vi "SINGLE_v15_5.vi"() -> ()   [LabVIEW 2017]
uses:
  BERTTA/x64/Debug/BERTTA.dll
panel:
  in  "Add comment":string
  in  "OK Button":bool
  out "Started:":string
  in  "SHUTDOWN":bool
  in  "MASTER CONTROL":bool
  in  "Tab Control":T1(tab)
  out "Output File":path caption="selected path"
  in  "Browse folder":path=path "C:/Users/shresplab/Desktop" caption="start path"
  in  "Read Seq":bool
  in  "Save Seq":bool
  in  "Configuration file":path caption="Filename"
  in  "OK Button 2":bool
  out "Boolean":bool
  in  "User (initials)":string
  in  "Project name":string
  in  "Description":string
  out "Led11 12":bool
  out "Target amount":dbl
  out "Scale weight":dbl
  out "Amount now":dbl
  out "Flow rate":dbl
  out "Time to target":dbl format="%<%H:%M:%S>t"
  out "Current step":dbl
  out "Target":dbl
  out "Amount now":dbl
  out "PUMP3":bool
  out "Led11 11":bool
  out "Amount now":dbl
  out "Target":dbl
  out "Current step":dbl
  out "Time to target":dbl format="%<%H:%M:%S>t"
  out "Flow rate":dbl
  out "Amount now":dbl
  out "Scale weight":dbl
  out "Target amount":dbl
  out "PUMP2":bool
  out "Target amount":dbl format="Target amount:        %#_g"
  out "Scale weight":dbl format="Scale weight:     %#_4g"
  out "Amount now":dbl format="Amount now:      %#_4g"
  out "Flow rate":dbl format="Flow rate:                   %#_4g"
  out "Time to target":dbl format="Time to target:     %<%H:%M:%S>t"
  out "Current step":dbl format="Current step:              %#_g"
  out "Target":dbl format="Target:                %#_4g"
  out "Amount now":dbl format="Amount now:    %#_4g"
  out "Led11 10":bool
  out "PUMP1":bool
  out "Sensor OK 6":bool
  out "Sensor OK 5":bool
  out "Sensor OK 4":bool
  out "Sensor OK 3":bool
  out "Tr":dbl format="Tr:              %#_4g"
  out "Tj in":dbl format="Tj in:        %#_4g"
  out "Tj out":dbl format="Tj out:        %#_4g"
  out "T set":dbl format="T set:          %#_4g"
  out "Current step":i32 format="Current step:  %.0f"
  out "RPM":dbl format="RPM:          %#_g"
  out "Torque 2":dbl format="Torque:      %#_g"
  out "T external 3":dbl format="T (S2):       %#_4g"
  out "Waveform Chart 5":dynamicdata(graph)
  out "Waveform Chart 6":dynamicdata(graph)
  out "Waveform Chart 7":dynamicdata(graph)
  in  "OK Button 11":bool=TRUE
  out "Table":string[][](table)=[["14.8.2017 18.06.59", "0,000000", "417,670000", "-0,150000", "1,000000", "22,220000", "23,366837", "23,574959", "23,985852", "23,690000", "240,000000", "4,000000", "0,000000", "397,000000", "-397,000000", "1,000000"], ["14.8.2017 18.07.06", "0,000000", "417,640000", "-0,120000", "1,000000", "22,220000", "23,763115", "23,906257", "23,985694", "23,680000", "240,000000", "4,000000", "0,000000", "397,000000", "-397,000000", "1,000000"], ["14.8.2017 18.07.13", "0,000000", "417,640000", "-0,120000", "1,000000", "22,220000", "23,965922", "24,013440", "23,984906", "23,670000", "240,000000", "4,100000", "3,000000", "397,000000", "-397,000000", "1,000000"], ["14.8.2017 18.07.21", "0,000000", "417,640000", "-0,120000", "1,000000", "22,220000", "23,943860", "23,900110", "23,987113", "23,670000", "240,000000", "4,000000", "0,000000", "397,000000", "-397,000000", "1,000000"], ["14.8.2017 18.07.28", "0,000000", "417,640000", "-0,120000", "1,000000", "22,220000", "23,736328", "23,600018", "23,989004", "23,660000", "240,000000", "4,000000", "0,000000", "397,000000", "-397,000000", "1,000000"], ["14.8.2017 18.07.36", "0,000000", "417,640000", "-0,120000", "1,000000", "22,220000", "23,480910", "23,324538", "23,991053", "23,660000", "240,000000", "4,000000", "0,000000", "397,000000", "-397,000000", "1,000000"], ["14.8.2017 18.07.43", "0,000000", "417,640000", "-0,120000", "2,000000", "22,220000", "23,195579", "23,008270", "23,999093", "23,650000", "240,000000", "4,000000", "0,000000", "397,000000", "-397,000000", "1,000000"], ["14.8.2017 18.07.51", "0,000000", "417,650000", "-417,650000", "1,000000", "22,220000", "22,862541", "22,649021", "24,003979", "23,650000", "240,000000", "4,000000", "0,000000", "397,000000", "-397,000000", "2,000000"], ["14.8.2017 18.07.58", "0,000000", "417,640000", "0,010000", "1,000000", "22,220000", "22,541353", "22,354878", "24,005398", "23,650000", "240,000000", "4,000000", "0,000000", "397,000000", "-397,000000", "1,000000"], ["14.8.2017 18.08.06", "0,000000", "417,640000", "0,010000", "1,000000", "22,220000", "22,347931", "22,253738", "24,007605", "23,640000", "240,000000", "4,100000", "0,000000", "397,000000", "-397,000000", "1,000000"], ["14.8.2017 18.08.13", "0,000000", "417,640000", "0,010000", "1,000000", "22,220000", "22,329030", "22,302102", "24,006028", "23,640000", "240,000000", "4,000000", "0,000000", "395,820000", "-395,820000", "1,000000"], ["14.8.2017 18.08.20", "0,000000", "417,640000", "0,010000", "1,000000", "22,220000", "22,466849", "22,511320", "24,002403", "23,630000", "240,000000", "4,000000", "0,000000", "395,830000", "-0,010000", "1,000000"], ["14.8.2017 18.08.28", "0,000000", "417,640000", "0,010000", "1,000000", "22,220000", "22,707062", "22,835101", "24,000984", "23,620000", "240,000000", "4,000000", "0,000000", "395,830000", "-0,010000", "1,000000"], ["14.8.2017 18.08.35", "0,000000", "417,640000", "0,010000", "1,000000", "22,220000", "23,054104", "23,232979", "24,001299", "23,600000", "240,000000", "4,000000", "0,000000", "395,830000", "-0,010000", "1,000000"], ["14.8.2017 18.08.43", "0,000000", "417,640000", "0,010000", "1,000000", "22,220000", "23,412371", "23,522793", "24,002560", "23,590000", "240,000000", "4,000000", "0,000000", "395,820000", "0,000000", "1,000000"], ["14.8.2017 18.08.51", "0,000000", "417,640000", "0,010000", "1,000000", "22,220000", "23,596247", "23,656125", "24,003821", "23,580000", "240,000000", "4,000000", "0,000000", "395,820000", "0,000000", "1,000000"]]
  out "LED_5":bool
  out "LED_4":bool
  in  "PAUSE/RUN 4":bool
  in  "TEMP RAMP":dbl[][](array[numeric])
  out "LED_3":bool
  out "LED_2":bool
  out "LED_1":bool
  out "LED_MANUAL":bool
  in  "Reset 6":bool
  in  "Manual/Ramp":bool=TRUE
  in  "Sensor selector":bool=TRUE
  in  "Tr/Tj mode selector":bool=TRUE
  out "LED STOP":bool
  in  "Failsafe":dbl=20.0 format="Failsafe temperature:            %#_g"
  out "Current temp":dbl format="Current temperature S1:       %#_4g"
  out "Sensor OK":bool
  out "T external 2":dbl format="Current temperature S2:       %#_4g"
  in  "OK Button 3":bool
  out "Waveform Chart":dynamicdata(graph)
  in  "X scales":i64(slide)=50 scale=0.0..100.0
  in  "PAUSE/RUN 9":bool=TRUE
  out "Led11 7":bool
  out "Led11 6":bool
  in  "PAUSE/RUN 3":bool
  in  "Tube select 3":u32(ring) items=["Big tube", "Double big tube", "Medium tube", "Small tube"]
  in  "Reset 8":bool
  out "Led11 9":bool
  in  "?":bool
  in  "Grams / min 3":dbl
  out "RPM 3":dbl format="%_4f"
  out "Flow rate (g/min) 3":dbl
  out "Scale reading 3":dbl
  out "Step amount now 3":dbl
  out "Total amount now 3":dbl
  out "Elapsed / step 3":dbl format="%<%H:%M:%S>t"
  out "Time to target 3":dbl format="%<%H:%M:%S>t"
  out "Led5 5":bool
  out "Led4 5":bool
  out "Led3 5":bool
  out "Led2 5":bool
  out "Led1 5":bool
  in  "PumpSeq 6":dbl[][](array[numeric])=[[0.0, 0.0, 0.0, 0.0, 0.0, 0.0, 0.0, 0.0, 0.0, 0.0], [0.0, 0.0, 0.0, 0.0, 0.0, 0.0, 0.0, 0.0, 0.0, 0.0], [0.0, 0.0, 0.0, 0.0, 0.0, 0.0, 0.0, 0.0, 0.0, 0.0], [0.0, 0.0, 0.0, 0.0, 0.0, 0.0, 0.0, 0.0, 0.0, 0.0], [0.0, 0.0, 0.0, 0.0, 0.0, 0.0, 0.0, 0.0, 0.0, 0.0], [0.0, 0.0, 0.0, 0.0, 0.0, 0.0, 0.0, 0.0, 0.0, 0.0], [0.0, 0.0, 0.0, 0.0, 0.0, 0.0, 0.0, 0.0, 0.0, 0.0], [0.0, 0.0, 0.0, 0.0, 0.0, 0.0, 0.0, 0.0, 0.0, 0.0], [0.0, 0.0, 0.0, 0.0, 0.0, 0.0, 0.0, 0.0, 0.0, 0.0], [0.0, 0.0, 0.0, 0.0, 0.0, 0.0, 0.0, 0.0, 0.0, 0.0]]
  out "Led11 8":bool
  in  "PAUSE/RUN 8":bool=TRUE
  out "Led11 7":bool
  out "Led11 6":bool
  in  "PAUSE/RUN 2":bool
  in  "Tube select 2":u32(ring) items=["Big tube", "Double big tube", "Medium tube", "Small tube"]
  out "Led11 7":bool
  in  "?":bool
  in  "Grams / min 2":dbl
  out "RPM 2":dbl format="%_4f"
  out "Flow rate (g/min) 2":dbl
  out "Scale reading 2":dbl
  out "Step amount now 2":dbl
  out "Total amount now 2":dbl
  out "Elapsed / step 2":dbl format="%<%H:%M:%S>t"
  out "Time to target 2":dbl format="%<%H:%M:%S>t"
  out "Led5 4":bool
  out "Led4 4":bool
  out "Led3 4":bool
  out "Led2 4":bool
  out "Led1 4":bool
  in  "PumpSeq 5":dbl[][](array[numeric])=[[0.0, 0.0, 0.0, 0.0, 0.0, 0.0, 0.0, 0.0, 0.0, 0.0], [0.0, 0.0, 0.0, 0.0, 0.0, 0.0, 0.0, 0.0, 0.0, 0.0], [0.0, 0.0, 0.0, 0.0, 0.0, 0.0, 0.0, 0.0, 0.0, 0.0], [0.0, 0.0, 0.0, 0.0, 0.0, 0.0, 0.0, 0.0, 0.0, 0.0], [0.0, 0.0, 0.0, 0.0, 0.0, 0.0, 0.0, 0.0, 0.0, 0.0], [0.0, 0.0, 0.0, 0.0, 0.0, 0.0, 0.0, 0.0, 0.0, 0.0], [0.0, 0.0, 0.0, 0.0, 0.0, 0.0, 0.0, 0.0, 0.0, 0.0], [0.0, 0.0, 0.0, 0.0, 0.0, 0.0, 0.0, 0.0, 0.0, 0.0], [0.0, 0.0, 0.0, 0.0, 0.0, 0.0, 0.0, 0.0, 0.0, 0.0], [0.0, 0.0, 0.0, 0.0, 0.0, 0.0, 0.0, 0.0, 0.0, 0.0]]
  out "Led11 6":bool
  in  "Reset 7":bool
  in  "PAUSE/RUN 7":bool=TRUE
  out "Led5 7":bool
  out "Led4 6":bool
  in  "PAUSE/RUN":bool
  in  "Tube select":u32(ring) items=["Big tube", "Double big tube", "Medium tube", "Small tube"]
  out "Led11 5":bool
  out "RPM":dbl format="RPM                      %_4f"
  out "Flow rate (g/min)":dbl format="Flow rate               %#_g"
  out "Scale reading":dbl format="Scale reading       %#_g"
  out "Step amount now":dbl format="Step amount       %#_g"
  out "Total amount now":dbl format="Total amount      %#_g"
  out "Elapsed / step":dbl format="Elapsed / step      %<%H:%M:%S>t"
  out "Time to target":dbl format="Time to target     %<%H:%M:%S>t"
  out "Led5 3":bool
  out "Led4 3":bool
  out "Led3 3":bool
  out "Led2 3":bool
  out "Led1 3":bool
  in  "PumpSeq 4":dbl[][](array[numeric])=[[0.0, 0.0, 0.0, 0.0, 0.0, 0.0, 0.0, 0.0, 0.0, 0.0], [0.0, 0.0, 0.0, 0.0, 0.0, 0.0, 0.0, 0.0, 0.0, 0.0], [0.0, 0.0, 0.0, 0.0, 0.0, 0.0, 0.0, 0.0, 0.0, 0.0], [0.0, 0.0, 0.0, 0.0, 0.0, 0.0, 0.0, 0.0, 0.0, 0.0], [0.0, 0.0, 0.0, 0.0, 0.0, 0.0, 0.0, 0.0, 0.0, 0.0], [0.0, 0.0, 0.0, 0.0, 0.0, 0.0, 0.0, 0.0, 0.0, 0.0], [0.0, 0.0, 0.0, 0.0, 0.0, 0.0, 0.0, 0.0, 0.0, 0.0], [0.0, 0.0, 0.0, 0.0, 0.0, 0.0, 0.0, 0.0, 0.0, 0.0], [0.0, 0.0, 0.0, 0.0, 0.0, 0.0, 0.0, 0.0, 0.0, 0.0], [0.0, 0.0, 0.0, 0.0, 0.0, 0.0, 0.0, 0.0, 0.0, 0.0]]
  in  "?":bool
  in  "Grams / min":dbl format="Manual g/min:  %#_g"
  out "Led11 4":bool
  in  "Reset 5":bool
  out "Waveform Chart 18":dynamicdata(graph)
  in  "OK Button 4":bool
  out "Waveform Chart 16":dynamicdata(graph)
  in  "OK Button 5":bool
  out "Waveform Chart 17":dynamicdata(graph)
  in  "OK Button 6":bool
  in  "PAUSE/RUN 5":bool
  in  "?":bool
  in  "Scale port":dbl=5.0
  out "Waveform Chart 15":dynamicdata(graph)
  in  "OK Button 8":bool
  in  "PAUSE/RUN 6":bool
  in  "Set RPM":i32
  in  "Remote / Manual":bool
  out "RPM":dbl
  out "Torque":dbl
  out "Waveform Chart 4":dynamicdata(graph)
  in  "OK Button 7":bool
  in  "CDAQ 1 Temp Control":tag="EASY9217_1"
  in  "CDAQ PAM Control":tag="EASY9747"
  in  "PORT PUMP2":i32 format="PUMP 2 PORT:  %.0f"
  in  "PORT PUMP3":i32 format="PUMP 3 PORT:  %.0f"
  in  "PORT PUMP1":i32 format="PUMP 1 PORT:  %.0f"
  in  "Save PortDev":bool
  in  "LAUDA":i32 format="LAUDA 1 PORT:  %.0f"
  in  "HEIDOLPH":i32 format="HEIDOLPH 1 PORT:  %.0f"
  in  "SCALE1":i32 format="SCALE 1 PORT:  %.0f"
  in  "SCALE2":i32 format="SCALE 2 PORT:  %.0f"
  in  "SCALE 3":i32 format="SCALE 3 PORT:  %.0f"
  # "Sensor:"
  # "Control:"
  # "PUMP & SCALE 3"
  # "STEP"
  # "TOTAL"
  # "PUMP & SCALE 2"
  # "STEP"
  # "TOTAL"
  # "PUMP & SCALE 1"
  # "STEP"
  # "TOTAL"
  # "MANUAL"
  # "RAMP"
  # "Temp Target       Time Target          Wait Time"
  # "STOP"
  # "g              min"
  # "g              min"
  # "g              min"
  # "PAM control"
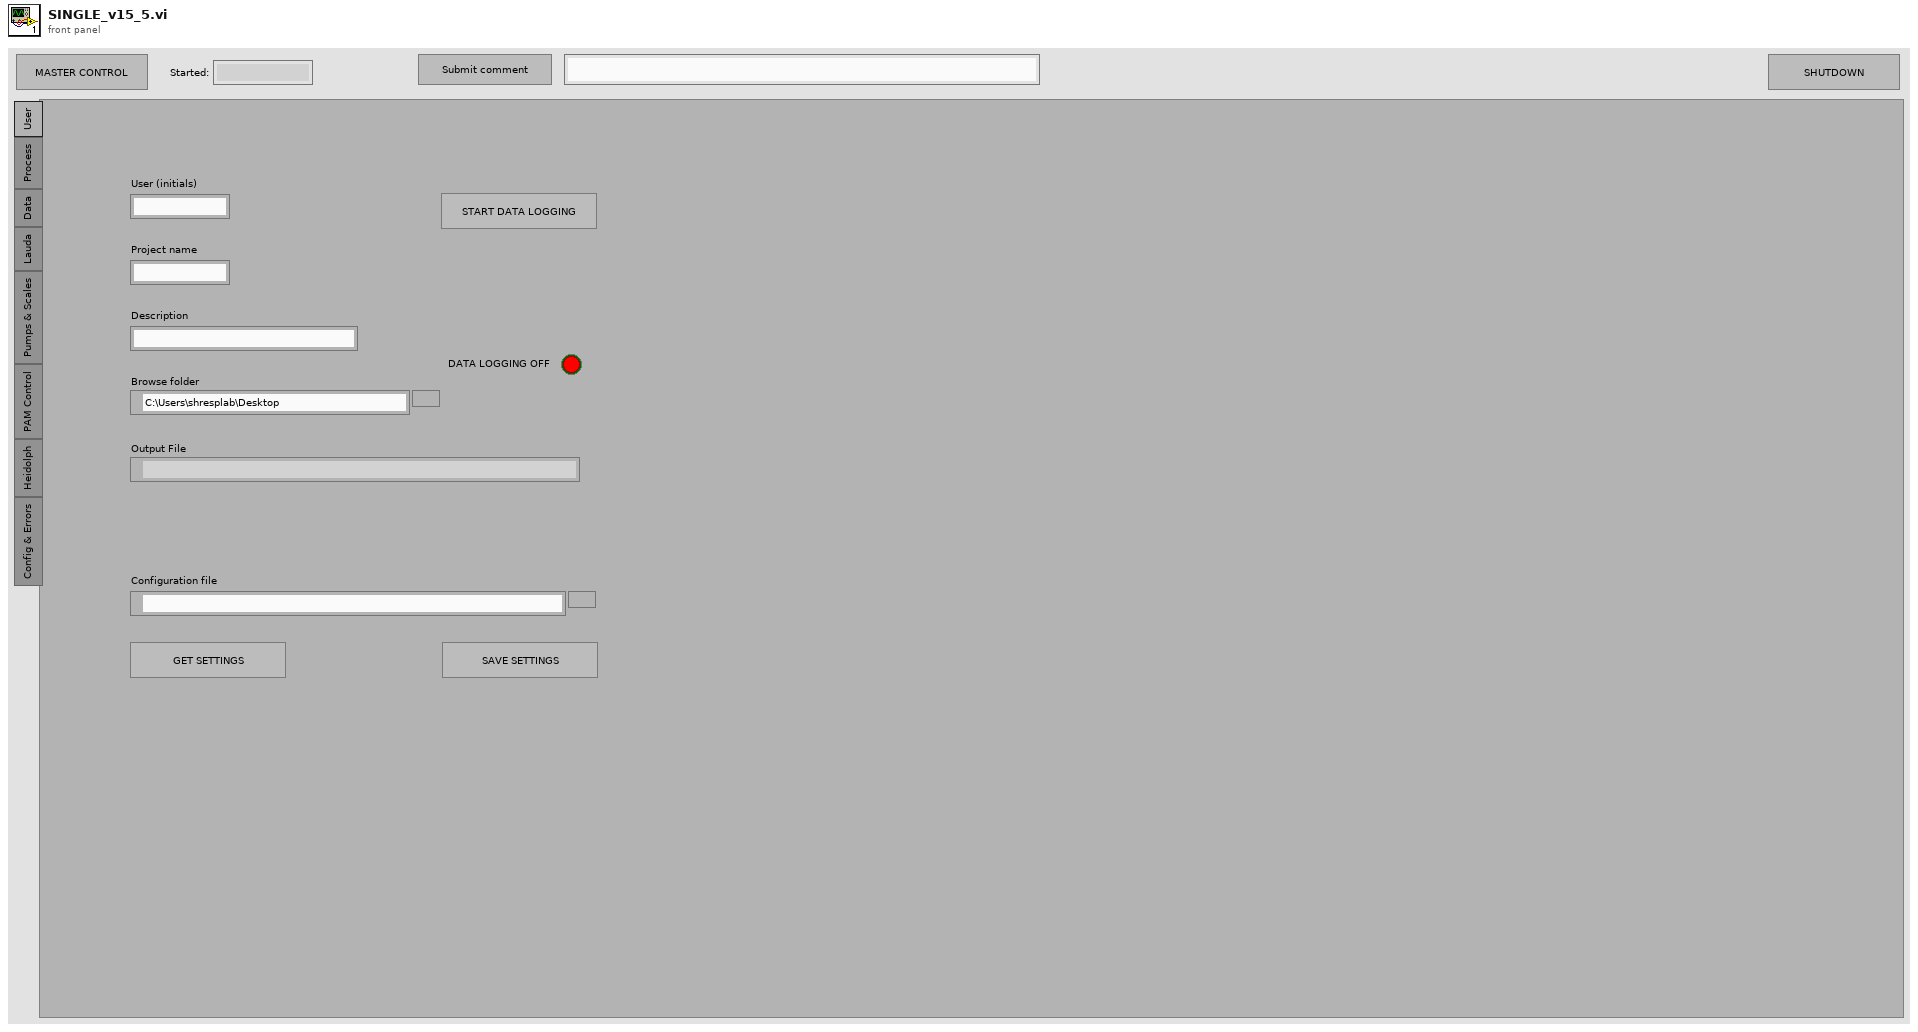
[diagram p1: front panel]
types:
  T1 = enum32{"User", "Process", "Data", "Lauda", "Pumps & Scales", "PAM Control", "Heidolph", "Config & Errors"}
diagram:
  n1 = while {
    i -> [w192]
    stop <- FALSE stop-if-true
    w126 = i64 1000 ("y")
    # "SCALE & PUMP 3"
    n2 = And(x="PAUSE/RUN 6", y="MASTER CONTROL") -> (x .and. y?=w116:bool)
    n3 = Not(x="MASTER CONTROL") -> (.not. x?=w227:bool)
    n4 = Boolean To (0,1)(Boolean="PAUSE/RUN 7") -> (0, 1=w12:i16)
    n5 = Boolean To (0,1)(Boolean="PAUSE/RUN 8") -> (0, 1=w11:i16)
    n6 = Boolean To (0,1)(Boolean="PAUSE/RUN 9") -> (0, 1=w10:i16)
    n7 = control-ref of="This VI"() -> (w112:refnum<vi>)
    n8 = Multiply(x="X scales", y=w126) -> (x*y=w127:i64)
    n9 = Boolean To (0,1)(Boolean=w227) -> (0, 1=w228:i16)
    n10 = call "RampCTRL_1.vi"("TEMP RAMP"="TEMP RAMP", "Reset 6"="Reset 6") -> ("Array"=w149:dbl[], "Array 2"=w150:dbl[], "Array 3"=w151:dbl[])  [unwired: 7 in]
    n11 = Add(x=w127, y=w126) -> (x+y=w32:i64)
    n12 = for {
      N: w228 -> [_]
      n13 = Get Date/Time String(want seconds? (F)=TRUE) -> (time string=→"Started:":string)  [unwired: 2 in, 1 out]
    }
    n14 = Select(t="Set RPM", s=w116, f=10) -> (s? t:f=w119:i32)
    n15 = Boolean To (0,1)(Boolean="Sensor selector") -> (0, 1=w144:i16)
    n16 = feedback #1() -> (w125:i64)  [unwired: 1 in]
    n17 = feedback-in #1(w32) -> ()
    n18 = call "shutdown sequence.vi"("SHUTDOWN"="SHUTDOWN", "VI in"=w112) -> ()  [unwired: 10 in]
    n19 = Boolean To (0,1)(Boolean="SHUTDOWN") -> (0, 1=w111:i16)
    n20 = Boolean To (0,1)(Boolean="Reset 6") -> (0, 1=w161:i16)
    n21 = Not Equal?(x=w125, y=w32) -> (x != y?=w124:bool)
    n22 = property on="Waveform Chart" class="WFChart (strict)"() -> ("History Data"=w129:dynamicdata[])  [unwired: 2 in, 2 out]
    n23 = Boolean To (0,1)(Boolean="SHUTDOWN") -> (0, 1=w113:i16)
    n24 = Boolean To (0,1)(Boolean=w124) -> (0, 1=w122:i16)
    n25 = Array Size(array=w129) -> (size(s)=w123:i32)
    n26 = call "ReadMoxa8.vi"("PORT 1"="LAUDA", "PORT 2"="HEIDOLPH", "PORT 3"="SCALE1", "PORT 4"="SCALE2", "PORT 5"="SCALE 3", "PORT 6"="PORT PUMP1", "PORT 7"="PORT PUMP2", "PORT 8"="PORT PUMP3", "enable1"=w12, "enable2"=w11, "enable3"=w10) -> ("params"=w14:dbl[])  [unwired: 8 in]
    n27 = call "HEI_CTRL.vi"("shutdown"=w113, "Set RPM"=w119, "Remote / Manual"="Remote / Manual", "port3"="HEIDOLPH") -> ()  [unwired: 8 in]
    n28 = Boolean To (0,1)(Boolean="Tr/Tj mode selector") -> (0, 1=w145:i16)
    n29 = call "SensorMode1.vi"("Numeric"=w144, "Numeric 2"=w145) -> ("Sensor OK 4"=→"Sensor OK 4":bool, "Sensor OK 5"=→"Sensor OK 5":bool, "Sensor OK 6"=→"Sensor OK 6":bool, "Sensor OK 3"=→"Sensor OK 3":bool)  [unwired: 6 in]
    n30 = for {
      N: w122 -> [_]
      tunnel: w123 -> [w241]
      tunnel: w32 -> [w240]
      n31 = Add(x=w241, y=w240) -> (x+y=w239:i64)
      n32 = property on="Waveform Chart" class="WFChart (strict)"("XScale.Maximum"=w239) -> ()  [unwired: 2 in, 2 out]
    }
    n33 = Boolean To (0,1)(Boolean="Manual/Ramp") -> (0, 1=w159:i16)
    n34 = And(x="MASTER CONTROL", y="PAUSE/RUN 4") -> (x .and. y?=w158:bool)
    n35 = Build Array("LAUDA", "HEIDOLPH", "SCALE1", "SCALE2", "SCALE 3", "PORT PUMP1", "PORT PUMP2", "PORT PUMP3") -> (w133:i32[])
    n36 = Boolean To (0,1)(Boolean=w158) -> (0, 1=w157:i16)
    n37 = call "LaudaDAQ.vi"("device name"="CDAQ 1 Temp Control") -> (1:"Tj out"=→"Tj out":dbl, "data"=w221:dynamicdata, "Sensor OK"=→"Sensor OK":bool, 4:"Tj out"=→"Tj in":dbl, "T external 2"=w115:dbl)  [unwired: 5 in, 1 out]
    "T external 2" <- w115
    "T external 3" <- w115
    n38 = call "Ramp_Lauda_v3.vi"("manual"=w159, "Tr_Tj"=w145, "shutdown"=w111, "S1_S2"=w144, "Tr"=w14, "T_fail"="Failsafe", "enable"=w157, "time_set"=w150, "reset"=w161, "time_wait"=w149, "T_S2"=w115, "port"="LAUDA", "T_sp"=w151) -> ("LED_1"=→"LED_1":bool, "LED_manual"=→"LED_MANUAL":bool, "LED_2"=→"LED_2":bool, "step"=w136:dbl, "LED_stop"=→"LED STOP":bool, "LED_3"=→"LED_3":bool, "LED 4"=→"LED_4":bool, "LED 5"=→"LED_5":bool, "setpoint"=w15:dbl, "Tr_out"=w156:dbl, "T int"=w155:dbl)  [unwired: 2 in, 2 out]
    "Tr" <- w156
    "T set" <- w15
    "Current temp" <- w156
    n39 = Boolean To (0,1)(Boolean="Save PortDev") -> (0, 1=w195:i16)
    n40 = for {
      N: w195 -> [_]
      tunnel: w133 -> [w287]
      tunnel: "Save PortDev" -> [w288]
      n41 = call "Convert to Dynamic Data"("Array"=w287) -> ("Dynamic Data Type"=w286:dynamicdata)  [unwired: 3 in]
      n42 = call "Write To Measurement File3"("Signals"=w286, "Reset"=w288) -> ()  [unwired: 15 in, 3 out]
    }
    n43 = Add(x=w136, y=1.0) -> (x+y=→"Current step":dbl)
    n44 = Merge Signals(w15, w156, w155, w221) -> (w22:dynamicdata)
    "Waveform Chart" <- w22
    "Waveform Chart 5" <- w22
    n45 = Less?(x=w192, y=1.0) -> (x < y?=w190:bool)
    n46 = call "HEI_Data_single.vi"("params"=w14) -> ("RPM"=→"RPM" →"RPM":dbl, "Dynamic Data"=w26:dynamicdata, "Torque 2"=→"Torque 2":dbl, "Waveform Chart 4"=→"Waveform Chart 4":dynamicdata, "Torque"=→"Torque":dbl, "Waveform Chart 6"=→"Waveform Chart 6":dynamicdata)  [unwired: 12 in, 1 out]
    n47 = Boolean To (0,1)(Boolean=w190) -> (0, 1=w191:i16)
    n48 = for {
      N: w191 -> [_]
      tunnel: w190 -> [w281]
      n49 = while {
        tunnel: [w284] -> w280
        tunnel: w281 -> [w282]
        stop <- w285 stop-if-true
        n50 = call "Read From Measurement File2"("Enable"=TRUE, "Reset"=w282) -> ("Signals"=w284:dynamicdata, "EOF?"=w285:bool)  [unwired: 4 in, 4 out]
      }
      n51 = call "Convert from Dynamic Data2"("Dynamic Data Type"=w280) -> ("Array"=w263:dbl[])  [unwired: 3 in]
      n52 = Index Array(array=w263, index=0) -> (element=w273:dbl)
      n53 = Index Array(array=w263, index=1) -> (element=w272:dbl)
      n54 = Index Array(array=w263, index=2) -> (element=w271:dbl)
      n55 = Index Array(array=w263, index=3) -> (element=w270:dbl)
      n56 = Index Array(array=w263, index=4) -> (element=w269:dbl)
      n57 = Index Array(array=w263, index=5) -> (element=w264:dbl)
      n58 = Index Array(array=w263, index=6) -> (element=w266:dbl)
      n59 = Index Array(array=w263, index=7) -> (element=w265:dbl)
      n60 = property on="LAUDA" class="DigNum (strict)"("Val(Sgnl)"=w273) -> ()  [unwired: 2 in, 2 out]
      n61 = property on="HEIDOLPH" class="DigNum (strict)"("Val(Sgnl)"=w272) -> ()  [unwired: 2 in, 2 out]
      n62 = property on="SCALE1" class="DigNum (strict)"("Val(Sgnl)"=w271) -> ()  [unwired: 2 in, 2 out]
      n63 = property on="SCALE2" class="DigNum (strict)"("Val(Sgnl)"=w270) -> ()  [unwired: 2 in, 2 out]
      n64 = property on="SCALE 3" class="DigNum (strict)"("Val(Sgnl)"=w269) -> ()  [unwired: 2 in, 2 out]
      n65 = property on="PORT PUMP1" class="DigNum (strict)"("Val(Sgnl)"=w264) -> ()  [unwired: 2 in, 2 out]
      n66 = property on="PORT PUMP2" class="DigNum (strict)"("Val(Sgnl)"=w266) -> ()  [unwired: 2 in, 2 out]
      n67 = property on="PORT PUMP3" class="DigNum (strict)"("Val(Sgnl)"=w265) -> ()  [unwired: 2 in, 2 out]
    }
    n68 = Boolean To (0,1)(Boolean="OK Button 3") -> (0, 1=w202:i16)
    n69 = for {
      N: w202 -> [_]
      n70 = property on="Waveform Chart" class="WFChart (strict)"("History Data"=dynamicdata[] []) -> ()  [unwired: 2 in, 2 out]
    }
    n71 = Boolean To (0,1)(Boolean="OK Button 4") -> (0, 1=w200:i16)
    n72 = for {
      N: w200 -> [_]
      n73 = property on="Waveform Chart 18" class="WFChart (strict)"("History Data"=dynamicdata[] []) -> ()  [unwired: 2 in, 2 out]
    }
    n74 = Boolean To (0,1)(Boolean="OK Button 5") -> (0, 1=w142:i16)
    n75 = for {
      N: w142 -> [_]
      n76 = property on="Waveform Chart 16" class="WFChart (strict)"("History Data"=dynamicdata[] []) -> ()  [unwired: 2 in, 2 out]
    }
    n77 = call "IsmaCTRL_single.vi"("FR_manual"="Grams / min", "tube selector"="Tube select", "Manual"="?", "Reset"="Reset 5", "Pause"="PAUSE/RUN", "Setpoint_W   /   Setpoint_T"="PumpSeq 4", "Enable"="MASTER CONTROL", "Scale"=w14) -> ("Boolean 9"=→"Led11 5" →"Led11 10":bool, "Boolean"=→"Led1 3":bool, "Boolean 2"=→"Led2 3":bool, "Total target"=→"Target":dbl, "Boolean 3"=→"Led3 3":bool, "Boolean 4"=→"Led4 3":bool, "lastAmount"=→"Step amount now":dbl, "step"=→"Current step":dbl, "Boolean 5"=→"Led5 3":bool, "Boolean 6"=→"Led4 6":bool, "Boolean 7"=→"Led5 7":bool, "FR"=w94:dbl, "RPM"=w18:dbl, "Weight"=w90:dbl, "elapsed"=→"Elapsed / step":dbl, "time_to_target"=→"Time to target" →"Time to target":dbl, "pumpCTRL"=w106:dbl, "Target_step"=→"Target amount":dbl, "Boolean 8"=w98:bool)  [unwired: 1 out]
    "Flow rate" <- w94
    "Scale weight" <- w90
    "Led11 4" <- w98
    "Scale reading" <- w90
    "Flow rate (g/min)" <- w94
    "RPM" <- w18
    n78 = Boolean To (0,1)(Boolean="OK Button 6") -> (0, 1=w140:i16)
    n79 = for {
      N: w140 -> [_]
      n80 = property on="Waveform Chart 17" class="WFChart (strict)"("History Data"=dynamicdata[] []) -> ()  [unwired: 2 in, 2 out]
    }
    n81 = Multiply(x=w90, y=-1.0 ("x")) -> (x*y=→"Amount now" →"Amount now" →"Total amount now":dbl)
    n82 = And(x="PAUSE/RUN", y=w98) -> (x .and. y?=w178:bool)
    n83 = feedback #2() -> (w179:bool)  [unwired: 1 in]
    n84 = feedback-in #2(w178) -> ()
    n85 = Greater?(x=w106, y=70.0) -> (0:→"PUMP1":bool)
    n86 = Not Equal?(x=w179, y=w178) -> (x != y?=w177:bool)
    n87 = Boolean To (0,1)(Boolean=w177) -> (0, 1=w176:i16)
    n88 = for {
      N: w176 -> [_]
      n89 = property on="PAUSE/RUN" class="Bool (strict)"("Val(Sgnl)"=FALSE ("Value (Signaling)")) -> ()  [unwired: 2 in, 2 out]
    }
    n90 = Merge Signals(w90, w94) -> (w143:dynamicdata)
    "Waveform Chart 18" <- w143
    n91 = Boolean To (0,1)(Boolean="OK Button 7") -> (0, 1=w198:i16)
    n92 = for {
      N: w198 -> [_]
      n93 = property on="Waveform Chart 4" class="WFChart (strict)"("History Data"=dynamicdata[] []) -> ()  [unwired: 2 in, 2 out]
    }
    n94 = call "IsmaCTRL_2_single.vi"("FR_manual"="Grams / min 2", "tube selector"="Tube select 2", "Manual"="?", "Reset"="Reset 7", "Pause"="PAUSE/RUN 2", "Setpoint_W   /   Setpoint_T"="PumpSeq 5", "Enable"="MASTER CONTROL", "Scale"=w14) -> ("Boolean 9"=→"Led11 7" →"Led11 11":bool, "Boolean"=→"Led1 4":bool, "Boolean 2"=→"Led2 4":bool, "Total target"=→"Target":dbl, "Boolean 3"=→"Led3 4":bool, "Boolean 4"=→"Led4 4":bool, "lastAmount"=→"Amount now" →"Step amount now 2":dbl, "step"=→"Current step":dbl, "Boolean 5"=→"Led5 4":bool, "Boolean 6"=→"Led11 6":bool, "Boolean 7"=→"Led11 7":bool, "FR"=w77:dbl, "RPM"=w17:dbl, "Weight"=w78:dbl, "elapsed"=→"Elapsed / step 2":dbl, "time_to_target"=→"Time to target" →"Time to target 2":dbl, "pumpCTRL"=w71:dbl, "Target_step"=→"Target amount":dbl, "Boolean 8"=w61:bool)  [unwired: 1 out]
    "Scale weight" <- w78
    "Flow rate" <- w77
    "Led11 6" <- w61
    "Scale reading 2" <- w78
    "Flow rate (g/min) 2" <- w77
    "RPM 2" <- w17
    n95 = Boolean To (0,1)(Boolean="OK Button 8") -> (0, 1=w185:i16)
    n96 = for {
      N: w185 -> [_]
      n97 = property on="Waveform Chart 15" class="WFChart (strict)"("History Data"=dynamicdata[] []) -> ()  [unwired: 2 in, 2 out]
    }
    n98 = Merge Signals(w78, w77) -> (w173:dynamicdata)
    "Waveform Chart 16" <- w173
    n99 = Multiply(x=w78, y=-1.0) -> (x*y=→"Amount now" →"Total amount now 2":dbl)
    n100 = And(x="PAUSE/RUN 2", y=w61) -> (x .and. y?=w171:bool)
    n101 = Greater?(x=w71, y=70.0) -> (0:→"PUMP2":bool)
    n102 = feedback #3() -> (w172:bool)  [unwired: 1 in]
    n103 = feedback-in #3(w171) -> ()
    n104 = Not Equal?(x=w172, y=w171) -> (x != y?=w170:bool)
    n105 = Boolean To (0,1)(Boolean=w170) -> (0, 1=w169:i16)
    n106 = for {
      N: w169 -> [_]
      n107 = property on="PAUSE/RUN 2" class="Bool (strict)"("Val(Sgnl)"=FALSE ("Value (Signaling)")) -> ()  [unwired: 2 in, 2 out]
    }
    n108 = call "IsmaCTRL_3_single.vi"("FR_manual"="Grams / min 3", "tube selector"="Tube select 3", "Manual"="?", "Reset"="Reset 8", "Pause"="PAUSE/RUN 3", "Setpoint_W   /   Setpoint_T"="PumpSeq 6", "Enable"="MASTER CONTROL", "Scale"=w14) -> ("Boolean 9"=→"Led11 9" →"Led11 12":bool, "Boolean"=→"Led1 5":bool, "Boolean 2"=→"Led2 5":bool, "Total target"=→"Target":dbl, "Boolean 3"=→"Led3 5":bool, "Boolean 4"=→"Led4 5":bool, "lastAmount"=→"Amount now" →"Step amount now 3":dbl, "step"=→"Current step":dbl, "Boolean 5"=→"Led5 5":bool, "Boolean 6"=→"Led11 6":bool, "Boolean 7"=→"Led11 7":bool, "FR"=w47:dbl, "RPM"=w16:dbl, "Weight"=w46:dbl, "elapsed"=→"Elapsed / step 3":dbl, "time_to_target"=→"Time to target" →"Time to target 3":dbl, "pumpCTRL"=w52:dbl, "Target_step"=→"Target amount":dbl, "Boolean 8"=w37:bool)  [unwired: 1 out]
    "Scale weight" <- w46
    "Flow rate" <- w47
    "Led11 8" <- w37
    "Scale reading 3" <- w46
    "Flow rate (g/min) 3" <- w47
    "RPM 3" <- w16
    n109 = call "WriteMoxa8.vi"("PORT LAUDA 1"="LAUDA", "DATA LAUDA 1"=w15, "enable2"=w11, "DATA ISMA 1"=w18, "DATA ISMA 2"=w17, "enable1"=w12, "PORT ISMA 1"="PORT PUMP1", "DATA ISMA 3"=w16, "PORT ISMA 2"="PORT PUMP2", "PORT ISMA 3"="PORT PUMP3", "enable3"=w10) -> ()  [unwired: 5 in]
    n110 = Multiply(x=w46, y=-1.0) -> (x*y=→"Amount now" →"Total amount now 3":dbl)
    n111 = Merge Signals(w90, w78, w46) -> (→"Waveform Chart 7":dynamicdata)
    n112 = Greater?(x=w52, y=70.0) -> (0:→"PUMP3":bool)
    n113 = And(x="MASTER CONTROL", y=w37) -> (x .and. y?=w164:bool)
    n114 = Merge Signals(w46, w47) -> (w166:dynamicdata)
    "Waveform Chart 17" <- w166
    n115 = feedback #4() -> (w165:bool)  [unwired: 1 in]
    n116 = feedback-in #4(w164) -> ()
    n117 = Not Equal?(x=w165, y=w164) -> (x != y?=w163:bool)
    n118 = Boolean To (0,1)(Boolean=w163) -> (0, 1=w162:i16)
    n119 = for {
      N: w162 -> [_]
      n120 = property on="PAUSE/RUN 3" class="Bool (strict)"("Val(Sgnl)"=FALSE ("Value (Signaling)")) -> ()  [unwired: 2 in, 2 out]
    }
    n121 = call "Convert to Dynamic Data6"() -> ("Dynamic Data Type"=w21:dynamicdata)  [unwired: 4 in]
    n122 = call "Convert to Dynamic Data4"("2D Array"="PumpSeq 6") -> ("Dynamic Data Type"=w208:dynamicdata)  [unwired: 3 in]
    n123 = call "Convert to Dynamic Data3"("2D Array"="PumpSeq 5") -> ("Dynamic Data Type"=w209:dynamicdata)  [unwired: 3 in]
    n124 = call "Convert to Dynamic Data2"("2D Array"="PumpSeq 4") -> ("Dynamic Data Type"=w211:dynamicdata)  [unwired: 3 in]
    n125 = Merge Signals(w21, w208, w209, w211) -> (w210:dynamicdata)
    n126 = Boolean To (0,1)(Boolean="Save Seq") -> (0, 1=w207:i16)
    n127 = for {
      N: w207 -> [_]
      tunnel: w210 -> [w320]
      tunnel: "Configuration file" -> [w321]
      tunnel: "Save Seq" -> [w319]
      n128 = call "Write To Measurement File2"("Signals"=w320, "Reset"=w319, "Filename"=w321) -> ()  [unwired: 14 in, 3 out]
    }
    n129 = Boolean To (0,1)(Boolean="Read Seq") -> (0, 1=w206:i16)
    n130 = for {
      N: w206 -> [_]
      tunnel: "Configuration file" -> [w306]
      tunnel: "Read Seq" -> [w305]
      n131 = while {
        tunnel: [w318] -> w314
        tunnel: w306 -> [w317]
        tunnel: w305 -> [w315]
        stop <- w316 stop-if-true
        n132 = call "Read From Measurement File"("Filename"=w317, "Reset"=w315) -> ("Signals"=w318:dynamicdata, "EOF?"=w316:bool)  [unwired: 4 in, 4 out]
      }
      n133 = call "Convert from Dynamic Data"("Dynamic Data Type"=w314) -> ("Array"=w309:dbl[][])  [unwired: 3 in]
      n134 = Array Subset(array=w309, index (row)=20 ("index"), length (row)=10 ("length")) -> (w302:dbl[][])  [unwired: 2 in]
      n135 = Array Subset(array=w309, index (row)=10 ("index"), length (row)=10 ("length")) -> (w303:dbl[][])  [unwired: 2 in]
      n136 = Array Subset(array=w309, index (row)=30 ("index"), length (row)=8 ("length")) -> (w304:dbl[][])  [unwired: 2 in]
      n137 = property on="PumpSeq 6" class="Arr (strict)"("Val(Sgnl)"=w303) -> ()  [unwired: 2 in, 2 out]
      n138 = property on="PumpSeq 4" class="Arr (strict)"("Val(Sgnl)"=w304) -> ()  [unwired: 2 in, 2 out]
      n139 = property on="PumpSeq 5" class="Arr (strict)"("Val(Sgnl)"=w302) -> ()  [unwired: 2 in, 2 out]
    }
    n140 = Merge Signals(w143, w173, w166) -> (w222:dynamicdata)
    n141 = Merge Signals(w22, w222, w26) -> (w188:dynamicdata)
    n142 = Boolean To (0,1)(Boolean="OK Button 11") -> (0, 1=w19:i16)
    n143 = for {
      N: w19 -> [_]
      tunnel: w188 -> [w233]
      n144 = call "Build Table"("Include time data"=TRUE, "Signals"=w233) -> ("Table"=w237:string[][])  [unwired: 3 in, 6 out]
      n145 = Delete From Array(array=w237, length=23, index (col)=0 ("index (row)")) -> (array with subset deleted=→"Table":string[][])  [unwired: 1 in, 1 out]
    }
    n146 = Boolean To (0,1)(Boolean="PAUSE/RUN 5") -> (0, 1=w147:i16)
    n147 = for {
      N: w147 -> [_]
      tunnel: "MASTER CONTROL" -> [w245]
      tunnel: "PAUSE/RUN 5" -> [w244]
      n148 = And(x=w244, y="?") -> (x .and. y?=w253:bool)
      n149 = dll-call lib="C:/Users/shresplab/OneDrive - Kemira Oyj/Documents/GitHub/Bertta/BERTTA/x64/Debug/BERTTA.dll" fn="mettler"("port"="Scale port", "msg"=1) -> ("return type"=w247:dbl)  [unwired: 5 in, 2 out]
      n150 = And(x=w245, y=w253) -> (x .and. y?=w250:bool)
      n151 = Initialize Array(FALSE, 1 ("dimension size")) -> (w252:bool[])
      n152 = Replace Array Subset(array=w252, new element=w250, index=0) -> (w249:bool[])
      n153 = call "Convert to Dynamic Data5"("Double"=w247) -> ("Dynamic Data Type"=→"Waveform Chart 15":dynamicdata)  [unwired: 3 in]
      n154 = call "DAQ Assistant"("data"=w249, "device name"="CDAQ PAM Control") -> ()  [unwired: 16 in, 2 out]
    }
    n155 = call "filenameparser_09.vi"("Description"="Description", "start path"="Browse folder", "Project name"="Project name", "User (initials)"="User (initials)", "OK Button in"="OK Button 2") -> ("appended path 2"=w196:path, "appended path"=w224:path)  [unwired: 4 in, 1 out]
    "Output File" <- w196
    n156 = Boolean To (0,1)(Boolean="OK Button") -> (0, 1=w223:i16)
    n157 = for {
      N: w223 -> [_]
      tunnel: w224 -> [w294]
      w298 = " " ("string")
      n158 = property on="Add comment" class="Str"("Val(Sgnl)"="" ("Value (Signaling)")) -> ()  [unwired: 2 in, 2 out]
      n159 = Get Date/Time String(want seconds? (F)=TRUE) -> (date string=w301:string, time string=w299:string)  [unwired: 2 in]
      n160 = Concatenate Strings(w301, w298, w299, w298, "Add comment") -> (w297:string)
      n161 = feedback #5() -> (w296:string[])  [unwired: 1 in]
      n162 = Build Array (concatenate)(w296, w297) -> (w295:string[])
      n163 = feedback-in #5(w295) -> ()
      n164 = Write to Text File(file (use dialog)=w294, text=w295) -> ()  [unwired: 2 in, 3 out]
    }
    n165 = call "Header Names TWIN.vi"("Dynamic Data"=w188) -> ("Signals Out"=w189:dynamicdata)  [unwired: 10 in]
    n166 = call "Write To Measurement File"("Signals"=w189, "Enable"="OK Button 2", "Filename"=w196) -> ()  [unwired: 14 in, 3 out]
    "Boolean" <- "OK Button 2"
  }
